vi "Allosense - File to AWS NoSQL Converter.vi"() -> ()   [LabVIEW 2020]
uses:
  <vilib>/Utility/miscctls.llb/LVDateTimeRec.ctl
  <vilib>/Utility/file.llb/Read Delimited Spreadsheet (string).vi
panel:
  out "Index":i32
  out "AWS CLI Response":string
  out "AWS CLI Command":string
  in  "File Format":T1(ring)
  out "Delimiter":string="\t"
  out "File Read":string[][](array[string])
  # "TEAM ALLOSENSE\nDatathon File to NoSQL Converter\n\nDeveloper: Roman Sandoval\nDate: 07/17/20"
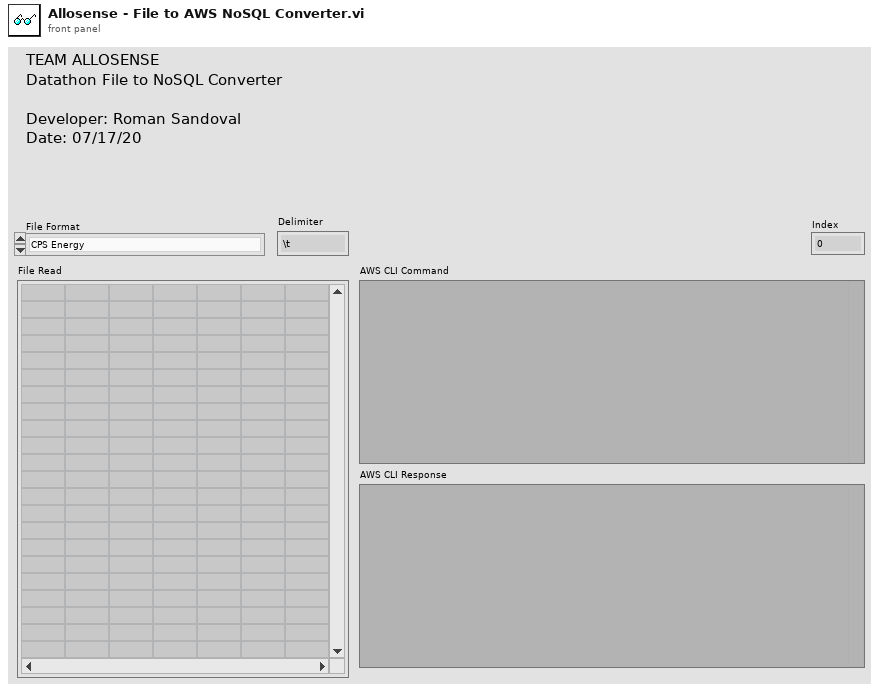
[diagram p1: front panel]
types:
  T1 = enum16{"CPS Energy", "San Antonio Water System", "TCEQ"}
  T2 = typedef "LVDateTimeRec.ctl" = cluster{"fractional second":dbl, "second":i32, "minute":i32, "hour":i32, "day of month":i32, "month":i32, "year":i32, "day of week":i32, "day of year":i32, "DST":i32}
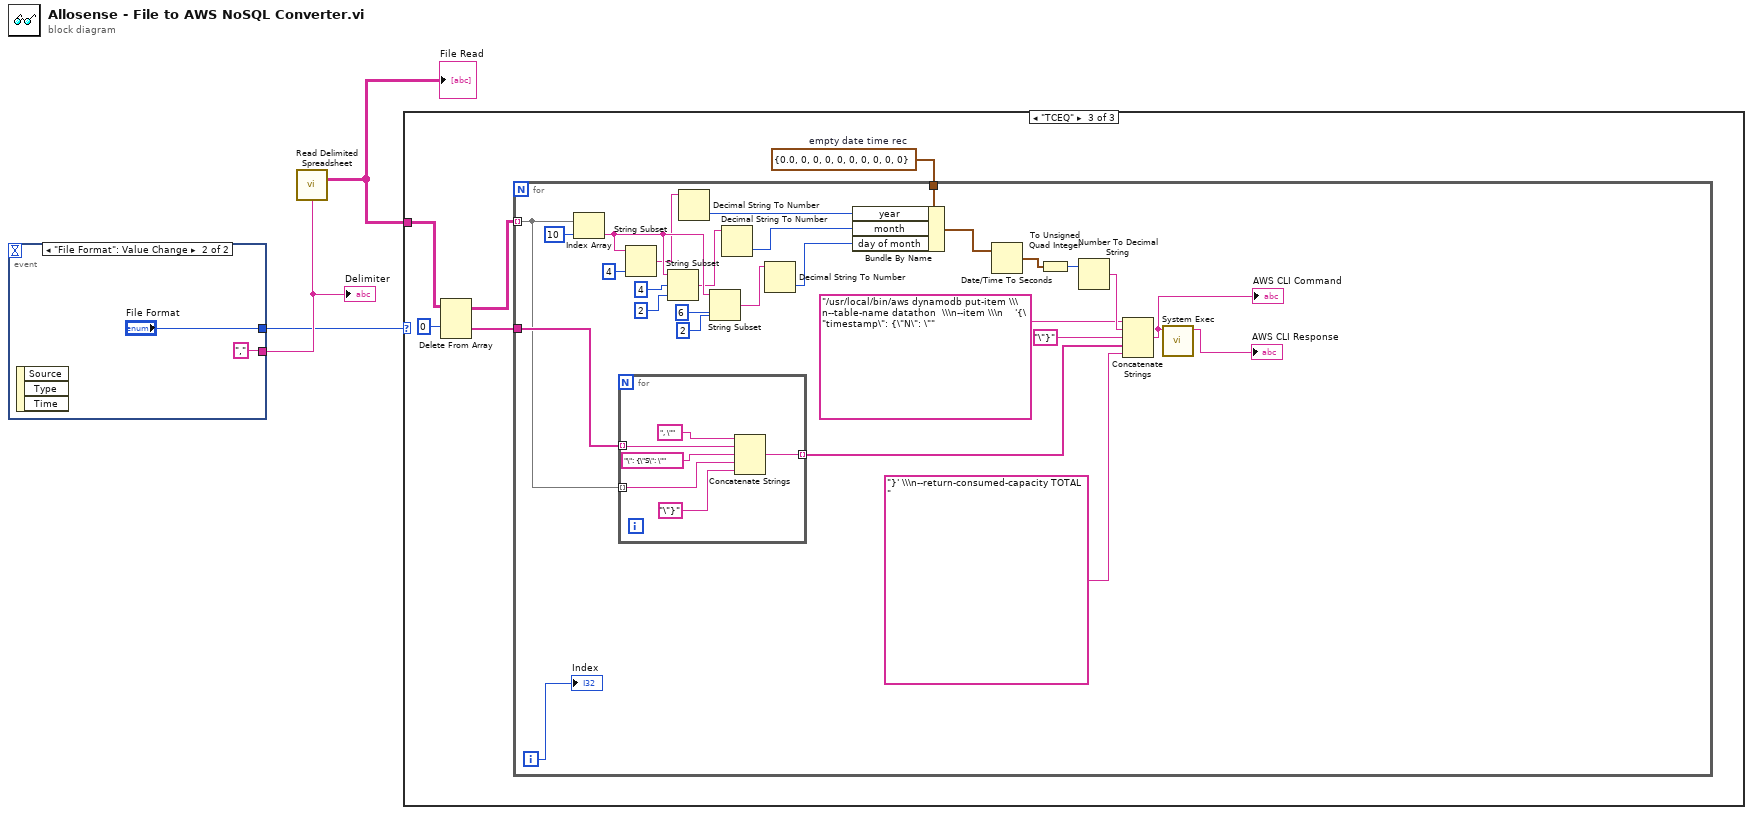
[diagram p0: block diagram]
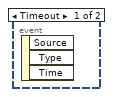
[diagram p4: hidden frame]
diagram:
  n1 = event shown="[1] \"File Format\": Value Change" {
    selector: _ -> [_ _]
    dyn-events: _ -> [_ _]
    timeout: _ -> [_ _]
    tunnel: [_ "File Format"] -> w2
    tunnel: [_ "," ("Delimiter")] -> w3
    event Timeout {
      n2 = event-data() -> ()  [unwired: 1 in, 3 out]
    }
    event "File Format": Value Change {
      n3 = event-data() -> ()  [unwired: 1 in, 3 out]
    }
  }
  "Delimiter" <- w3
  n4 = call-poly <vilib>:"Read Delimited Spreadsheet.vi"("delimiter (\\t)"=w3) -> ("all rows"=w1:string[][])  [unwired: 9 in, 5 out]
  "File Read" <- w1
  n5 = case shown="\"TCEQ\"" w2 {
    tunnel: w1 -> [_ _ w9]
    frame "CPS Energy", Default {
    }
    frame "San Antonio Water System" {
    }
    frame "TCEQ" {
      w7 = T2 {"fractional second"=0.0, "second"=0, "minute"=0, "hour"=0, "day of month"=0, "month"=0, "year"=0, "day of week"=0, "day of year"=0, "DST"=0}  # empty date time rec
      n6 = Delete From Array(array=w9, index (row)=0) -> (deleted portion=w8:string[], array with subset deleted=w6:string[][])  [unwired: 2 in]
      n7 = for {
        tunnel: w6 -> [w14] mode=indexing
        tunnel: w8 -> [w15]
        tunnel: w7 -> [w36]
        i -> [w16]
        n8 = Index Array(array=w14, index=10) -> (element=w32:string)
        n9 = for {
          tunnel: w15 -> [w42] mode=indexing
          tunnel: w14 -> [w40] mode=indexing
          tunnel: [w38] -> w11 mode=indexing
          (unwired) "\": {\"S\": \"" ("string")
          n10 = Concatenate Strings(", \"" ("command line"), w42, "\": {\"S\": \"" ("string"), w40, "\"}" ("string")) -> (w38:string)
        }
        n11 = String Subset(string=w32, length (rest)=4 ("length (rest)")) -> (substring=w29:string)  [unwired: 1 in]
        n12 = String Subset(string=w32, offset (0)=4 ("length (rest)"), length (rest)=2 ("length (rest)")) -> (substring=w28:string)
        n13 = Decimal String To Number(string=w29) -> (number=w26:i32)  [unwired: 2 in, 1 out]
        n14 = String Subset(string=w32, offset (0)=6, length (rest)=2 ("length (rest)")) -> (substring=w27:string)
        n15 = Decimal String To Number(string=w28) -> (number=w25:i32)  [unwired: 2 in, 1 out]
        n16 = Decimal String To Number(string=w27) -> (number=w24:i32)  [unwired: 2 in, 1 out]
        n17 = Bundle By Name(cluster=w36, "year"=w26, "month"=w25, "day of month"=w24) -> (w23:T2)
        n18 = Date/Time To Seconds(2:w23) -> (0:w19:timestamp)  [unwired: 1 in]
        n19 = To Unsigned Quad Integer(1:w19) -> (0:w22:u64)
        n20 = Number To Decimal String(number=w22) -> (decimal integer string=w21:string)  [unwired: 1 in]
        n21 = Concatenate Strings("/usr/local/bin/aws dynamodb put-item \\\n--table-name datathon  \\\n--item \\\n    '{\"timestamp\": {\"N\": \"" ("command line"), w21, "\"}" ("command line"), w11, "}' \\\n--return-consumed-capacity TOTAL  " ("command line")) -> (w18:string)
        "AWS CLI Command" <- w18
        n22 = call <vilib>:"System Exec.vi"("command line"=w18) -> ("standard output"=→"AWS CLI Response":string)  [unwired: 7 in, 3 out]
        "Index" <- w16
      }
    }
  }
